vi "test.vi"() -> ()   [LabVIEW 2013]
panel:
  out "subarray 2":dbl[](array[numeric])
  out "subarray":dbl[](array[numeric])
  out "sqrt(x)":dbl
  in  "array":dbl[][](array[numeric])=[[0.0, 0.0, 0.0]]
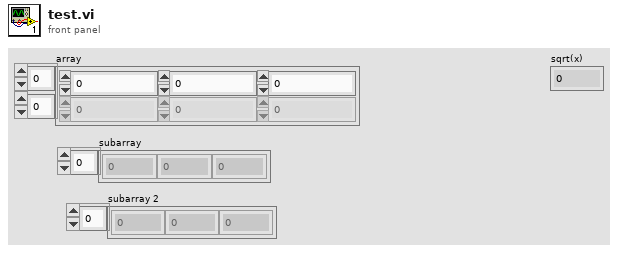
[diagram p1: front panel]
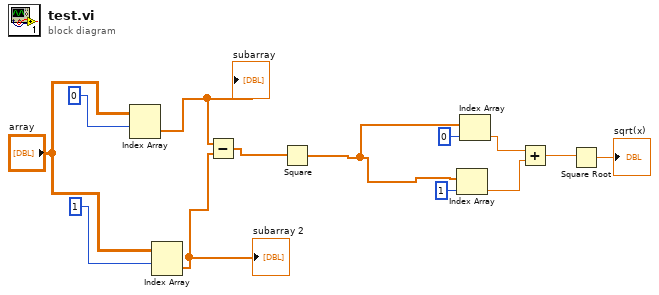
[diagram p0: block diagram]
diagram:
  n1 = Index Array(array="array", index (row)=0 ("index")) -> (element=w4:dbl[])  [unwired: 1 in]
  "subarray" <- w4
  n2 = Index Array(array="array", index (row)=1 ("index")) -> (element=w5:dbl[])  [unwired: 1 in]
  "subarray 2" <- w5
  n3 = Subtract(x=w4, y=w5) -> (x-y=w13:dbl[])
  n4 = Square(x=w13) -> (x^2=w10:dbl[])
  n5 = Index Array(array=w10, index=1) -> (element=w8:dbl)
  n6 = Index Array(array=w10, index=0) -> (element=w9:dbl)
  n7 = Add(x=w9, y=w8) -> (x+y=w7:dbl)
  n8 = Square Root(x=w7) -> (sqrt(x)=→"sqrt(x)":dbl)
